vi "Pobranie odległości do punktu docelowego z listy współrzędnych.vi"(10 "Lista współrzędnych":string[][](array[string]), 11 "Numer pobranego punktu":i32) -> (2 "Dojazd do punktu":string, 3 "Odl. do punktu docelowego":cluster{"X/E [m]":dbl, "Y/N [m]":dbl})   [LabVIEW 2015, in "Biblioteka moduł map v3.lvlib" / "Pomocnicze.lvlib"]
doc: "Pobranie z listy współrzędnych odległości do punktu docelowego od startu na podstawie numeru wiersza listy współrzędnych. W przypadku podania zbyd dużej wartości numeru pobranego wiersza wartość odległości od startu ustawiana jest na 0m w kierunku X i Y."
uses:
  Pomocnicze.lvlib
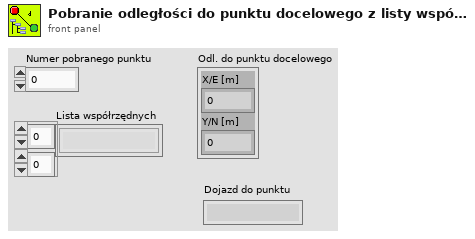
[diagram p1: front panel]
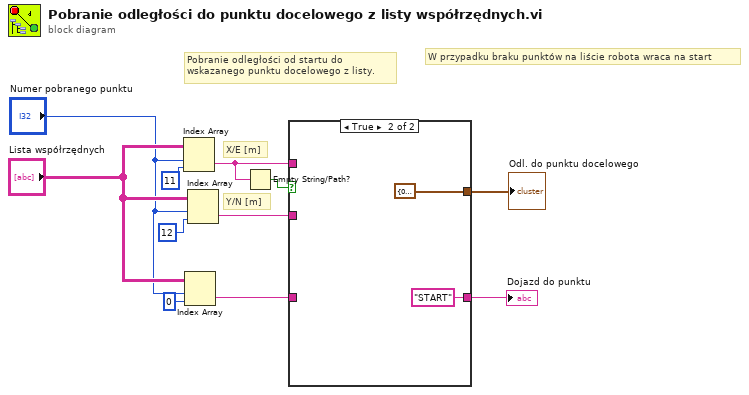
[diagram p0: block diagram]
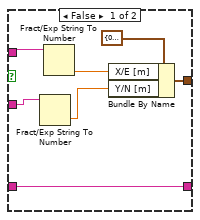
[diagram p2: hidden frame]
diagram:
  # "W przypadku braku punktów na liście robota wraca na start"
  # "Pobranie odległości od startu do\nwskazanego punktu docelowego z listy."
  # "Y/N [m]"
  # "X/E [m]"
  n1 = Index Array(array="Lista współrzędnych", index (row)="Numer pobranego punktu", index (col)=11 ("disabled index (col)")) -> (element=w10:string)
  n2 = Index Array(array="Lista współrzędnych", index (row)="Numer pobranego punktu", index (col)=0 ("disabled index (col)")) -> (element=w3:string)
  n3 = Index Array(array="Lista współrzędnych", index (row)="Numer pobranego punktu", index (col)=12 ("index (row)")) -> (element=w7:string)
  n4 = Empty String/Path?(string/path=w10) -> (empty?=w11:bool)
  n5 = case shown="True" w11 {
    tunnel: w10 -> [w16 _]
    tunnel: w7 -> [w15 _]
    tunnel: [w17 cluster{"X/E [m]":dbl, "Y/N [m]":dbl} {"X/E [m]"=0.0, "Y/N [m]"=0.0} ("Położenie")] -> w8
    tunnel: [w12 "START"] -> w2
    tunnel: w3 -> [w12 _]
    frame False {
      n6 = Fract/Exp String To Number(string=w15) -> (number=w14:dbl)  [unwired: 3 in, 1 out]
      n7 = Fract/Exp String To Number(string=w16) -> (number=w13:dbl)  [unwired: 3 in, 1 out]
      n8 = Bundle By Name(cluster=cluster{"X/E [m]":dbl, "Y/N [m]":dbl} {"X/E [m]"=0.0, "Y/N [m]"=0.0} ("Położenie"), "X/E [m]"=w13, "Y/N [m]"=w14) -> (w17:cluster{"X/E [m]":dbl, "Y/N [m]":dbl})
    }
    frame True {
    }
  }
  "Odl. do punktu docelowego" <- w8
  "Dojazd do punktu" <- w2
